vi "SubEvnts.vi"(8 "error in (no error)":errorcluster, 11 "SALCommunicatorView in":refnum<class "SALCommunicatorView.lvclass">) -> (0 "error out":errorcluster, 3 "SALCommunicatorView out":refnum<class "SALCommunicatorView.lvclass">)   [LabVIEW 2016, in "SALCommunicatorView.lvclass"]
uses:
  SALCommunicatorView.lvclass
  ts_sallv_exa/SALLV_EXA.lvlib
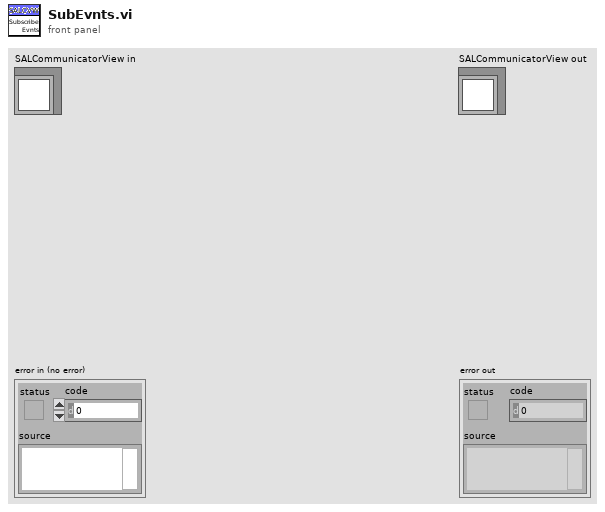
[diagram p1: front panel]
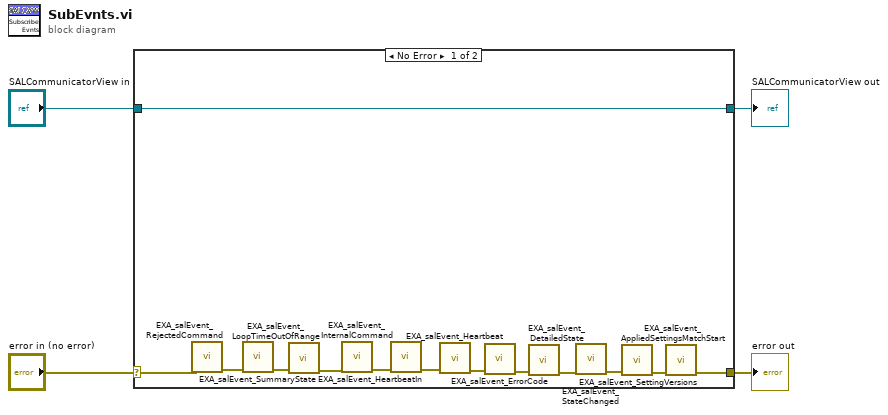
[diagram p0: block diagram]
diagram:
  n1 = case shown="No Error" "error in (no error)" {
    selector: "error in (no error)" -> [w16 w19]
    tunnel: [w5 w19] -> w3
    tunnel: [w17 w18] -> w1
    tunnel: "SALCommunicatorView in" -> [w17 w18]
    frame No Error {
      n2 = call "EXA_salEvent_RejectedCommand.vi"("error in (no error)"=w16) -> ("error out"=w15:errorcluster)  [unwired: 9 in, 1 out]
      n3 = call "EXA_salEvent_SummaryState.vi"("error in (no error)"=w15) -> ("error out"=w14:errorcluster)  [unwired: 9 in, 1 out]
      n4 = call "EXA_salEvent_LoopTimeOutOfRange.vi"("error in (no error)"=w14) -> ("error out"=w13:errorcluster)  [unwired: 9 in, 1 out]
      n5 = call "EXA_salEvent_InternalCommand.vi"("error in (no error)"=w13) -> ("error out"=w12:errorcluster)  [unwired: 9 in, 1 out]
      n6 = call "EXA_salEvent_HeartbeatIn.vi"("error in (no error)"=w12) -> ("error out"=w11:errorcluster)  [unwired: 9 in, 1 out]
      n7 = call "EXA_salEvent_Heartbeat.vi"("error in (no error)"=w11) -> ("error out"=w10:errorcluster)  [unwired: 9 in, 1 out]
      n8 = call "EXA_salEvent_ErrorCode.vi"("error in (no error)"=w10) -> ("error out"=w9:errorcluster)  [unwired: 9 in, 1 out]
      n9 = call "EXA_salEvent_DetailedState.vi"("error in (no error)"=w9) -> ("error out"=w8:errorcluster)  [unwired: 9 in, 1 out]
      n10 = call "EXA_salEvent_StateChanged.vi"("error in (no error)"=w8) -> ("error out"=w7:errorcluster)  [unwired: 9 in, 1 out]
      n11 = call "EXA_salEvent_AppliedSettingsMatchStart.vi"("error in (no error)"=w7) -> ("error out"=w6:errorcluster)  [unwired: 9 in, 1 out]
      n12 = call "EXA_salEvent_SettingVersions.vi"("error in (no error)"=w6) -> ("error out"=w5:errorcluster)  [unwired: 9 in, 1 out]
    }
    frame Error {
    }
  }
  "error out" <- w3
  "SALCommunicatorView out" <- w1
